vi "Init4VictorDrive.vi"(10 "Drive.lvclass 2":refnum<class "Drive.lvclass">) -> ()   [LabVIEW 2017, in "Drive.lvclass"]
uses:
  Drive.lvclass
  <vilib>/Rock Robotics/WPI/SafetyOutput/WPI_SafetyOutputConfigMenu.ctl
  Drive.lvclass/Drive.ctl
  <vilib>/Rock Robotics/WPI/RobotDrive/WPI_RobotDriveOpen4MotorWithExistingMotors.vi
panel:
  out "Drive.lvclass":refnum<class "Drive.lvclass">
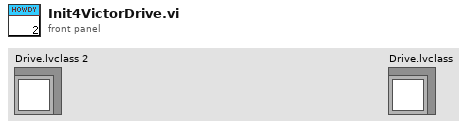
[diagram p1: front panel]
types:
  T1 = typedef "WPI_SafetyOutputConfigMenu.ctl" = enum16{"Enable", "Disable"}
  T2 = typedef "WPI_MotorControlDeviceRef.ctl" = cluster{"DeviceStatus":errorcluster, "Type":T3, "PWM":cluster{"PWM Channel":T4, "DeadBand":T5}, "CAN":cluster{"Device Number":u8, "SetOutput VI Ref":variant, "GetOutput VI Ref":variant, "Enable VI Ref":variant, "Disable VI Ref":variant, "Data":variant}, "Invert":bool, "DIO PWM":cluster{"PWM \"Enable\" Channel":T4, "DIOChannel":T6, "PWM Rate":dbl}}
  T3 = typedef "WPI_MotorControlType.ctl" = enum16{"PWM", "CAN", "DIO PWM"}
  T4 = typedef "FPGA_DIOPWMChannel.ctl" = enum8{"PWM 0", "PWM 1", "PWM 2", "PWM 3", "PWM 4", "PWM 5", "PWM 6", "PWM 7", "PWM 8", "PWM 9", "PWM MXP 0", "PWM MXP 1", "PWM MXP 2", "PWM MXP 3", "PWM MXP 4", "PWM MXP 5", "PWM MXP 6", "PWM MXP 7", "PWM MXP 8", "PWM MXP 9", "Invalid"}
  T5 = typedef "WPI_PWMDeadband.ctl" = cluster{"Name":string, "maxPositivePwm":i32, "minPositivePwm":i32, "centerPwm":i32, "maxNegativePwm":i32, "minNegativePwm":i32, "angularRange":u16}
  T6 = typedef "FPGA_DIOChannel.ctl" = enum8{"DIO 0", "DIO 1", "DIO 2", "DIO 3", "DIO 4", "DIO 5", "DIO 6", "DIO 7", "DIO 8", "DIO 9", "DIO MXP 0", "DIO MXP 1", "DIO MXP 2", "DIO MXP 3", "DIO MXP 4", "DIO MXP 5", "DIO MXP 6", "DIO MXP 7", "DIO MXP 8", "DIO MXP 9", "DIO MXP 10", "DIO MXP 11", "DIO MXP 12", "DIO MXP 13", "DIO MXP 14", "DIO MXP 15", "SPI Port CS1", "SPI Port CS2", "SPI Port CS3", "SPI Port MISO", "SPI Port MOSI", "Invalid"}
  T7 = typedef "WPI_RobotDriveDevRef.ctl" = cluster{"DevStatus":errorcluster, "Motors[]":T2[], "Square Inputs":bool, "Max Output":dbl}
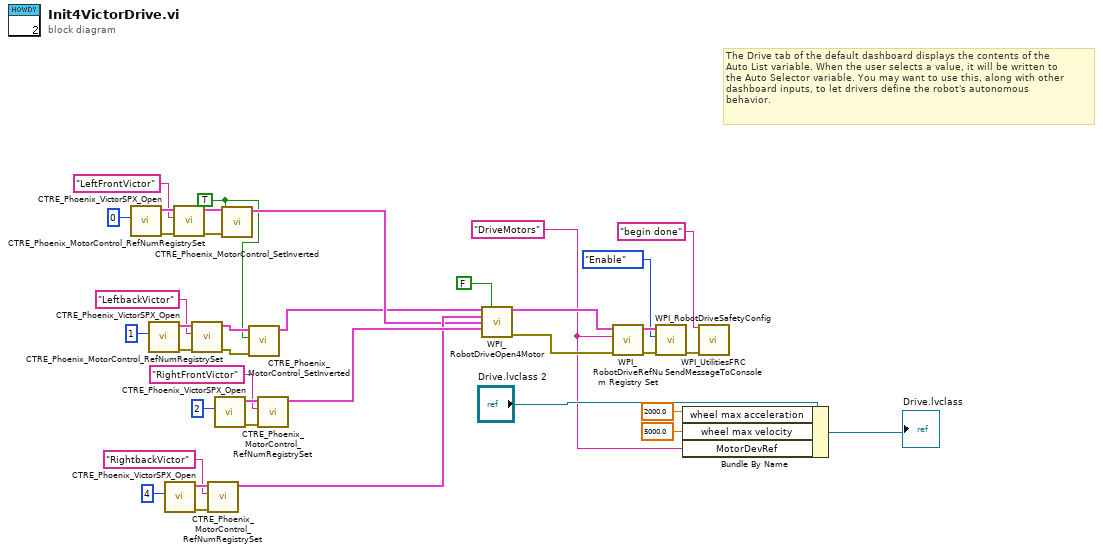
[diagram p0: block diagram]
diagram:
  w10 = "DriveMotors" ("refnum name")
  w2 = TRUE ("Invert?")
  # "The Drive tab of the default dashboard displays the contents of the\nAuto List variable. When the user selects a value, it will be written to\nthe Auto Selector variable. You may want to use this, along with other\ndashboard inputs, to let drivers define the robot's autonomous\nbehavior."
  n1 = call <vilib>:"CTRE_Phoenix_VictorSPX_Open.vi"("Device Number"=u8 0) -> ("error out"=w36:errorcluster, "CAN Talon SRX Ref"=w37:T2)  [unwired: 9 in]
  n2 = call <vilib>:"CTRE_Phoenix_VictorSPX_Open.vi"("Device Number"=u8 1) -> ("error out"=w24:errorcluster, "CAN Talon SRX Ref"=w25:T2)  [unwired: 9 in]
  n3 = call <vilib>:"CTRE_Phoenix_VictorSPX_Open.vi"("Device Number"=u8 4) -> ("error out"=w28:errorcluster, "CAN Talon SRX Ref"=w29:T2)  [unwired: 9 in]
  n4 = call <vilib>:"CTRE_Phoenix_MotorControl_RefNumRegistrySet.vi"("error in (no error)"=w36, "refnum name"="LeftFrontVictor", "PhoenixMotorControlDevRef"=w37) -> ("error out"=w22:errorcluster, "PhoenixMotorControlDevRef"=w21:T2)  [unwired: 7 in]
  n5 = call <vilib>:"CTRE_Phoenix_MotorControl_RefNumRegistrySet.vi"("error in (no error)"=w24, "refnum name"="LeftbackVictor", "PhoenixMotorControlDevRef"=w25) -> ("error out"=w5:errorcluster, "PhoenixMotorControlDevRef"=w4:T2)  [unwired: 7 in]
  n6 = call <vilib>:"CTRE_Phoenix_MotorControl_RefNumRegistrySet.vi"("error in (no error)"=w28, "refnum name"="RightbackVictor", "PhoenixMotorControlDevRef"=w29) -> ("PhoenixMotorControlDevRef"=w19:T2)  [unwired: 7 in, 1 out]
  n7 = call <vilib>:"CTRE_Phoenix_VictorSPX_Open.vi"("Device Number"=u8 2) -> ("error out"=w32:errorcluster, "CAN Talon SRX Ref"=w33:T2)  [unwired: 9 in]
  n8 = call <vilib>:"CTRE_Phoenix_MotorControl_SetInverted.vi"("error in (no error)"=w22, "Invert?"=w2, "PhoenixMotorControlDevRef"=w21) -> ("PhoenixMotorControlDevRef"=w6:T2)  [unwired: 7 in, 1 out]
  n9 = call <vilib>:"CTRE_Phoenix_MotorControl_SetInverted.vi"("error in (no error)"=w5, "Invert?"=w2, "PhoenixMotorControlDevRef"=w4) -> ("PhoenixMotorControlDevRef"=w3:T2)  [unwired: 7 in, 1 out]
  n10 = call <vilib>:"CTRE_Phoenix_MotorControl_RefNumRegistrySet.vi"("error in (no error)"=w32, "refnum name"="RightFrontVictor", "PhoenixMotorControlDevRef"=w33) -> ("PhoenixMotorControlDevRef"=w20:T2)  [unwired: 7 in, 1 out]
  n11 = call-poly <vilib>:"WPI_RobotDriveOpen4Motor.vi"("Rear Left Motor Dev Ref"=w3, "Square Inputs"=FALSE, "Rear Right Motor Dev Ref"=w19, "Front Left Motor Dev Ref"=w6, "Front Right Motor Dev Ref"=w20) -> ("RobotDriveDevRef"=w15:T7, "error out"=w14:errorcluster)  [unwired: 9 in]
  n12 = call <vilib>:"WPI_RobotDriveRefNum Registry Set.vi"("error in (no error)"=w14, "refnum name"=w10, "RobotDriveDevRef"=w15) -> ("error out"=w13:errorcluster, "RobotDriveDevRef"=w17:T7)  [unwired: 7 in]
  n13 = call <vilib>:"WPI_RobotDriveSafetyConfig.vi"("error in (no error)"=w13, "mode"=WPI_SafetyOutputConfigMenu."Enable", "RobotDriveDevRef"=w17) -> ("error out"=w12:errorcluster)  [unwired: 7 in, 1 out]
  n14 = Bundle By Name(cluster="Drive.lvclass 2", "wheel max acceleration"=2000.0, "wheel max velocity"=5000.0, "MotorDevRef"=w10) -> (→"Drive.lvclass":refnum<class "Drive.lvclass">)
  n15 = call <vilib>:"WPI_UtilitiesFRC SendMessageToConsole.vi"("Message"="begin done", "error in (no error)"=w12) -> ()  [unwired: 13 in, 1 out]
